vi "svx_Harmonic Generator.vi"(4 "noise amplitude":dbl=1.0 format="%.2f", 5 "# of harmonics":i32=5, 6 "sampling info":cluster{"Fs":dbl, "#s":dbl}={"Fs"=51200.0, "#s"=1024.0} {"#s" format="%.2p"; "Fs" format="%.2p"}, 7 "harmonics":T1(ring), 8 "error in (no error)":errorcluster, 9 "phase":dbl format="%.2f", 10 "Amplitude":dbl format="%.2f", 11 "fundamental":dbl format="%.2f") -> (0 "error out":errorcluster, 3 "Waveform":waveform(dbl))   [LabVIEW 2017]
uses:
  <vilib>/measure/maUtilsandCtls.llb/ma_Updatet0 DBL.vi
  <vilib>/measure/NI_MABase.lvlib
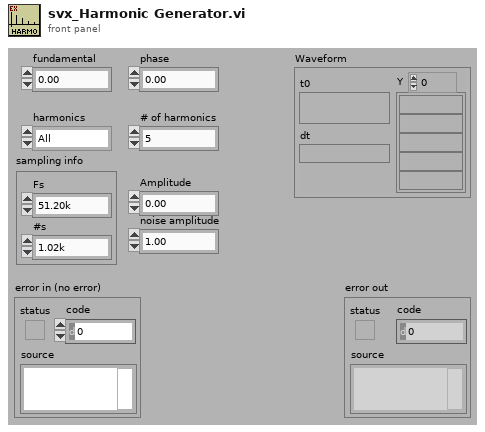
[diagram p1: front panel]
types:
  T1 = enum16{"All", "odd only", "even only", "Custom frequencies"}
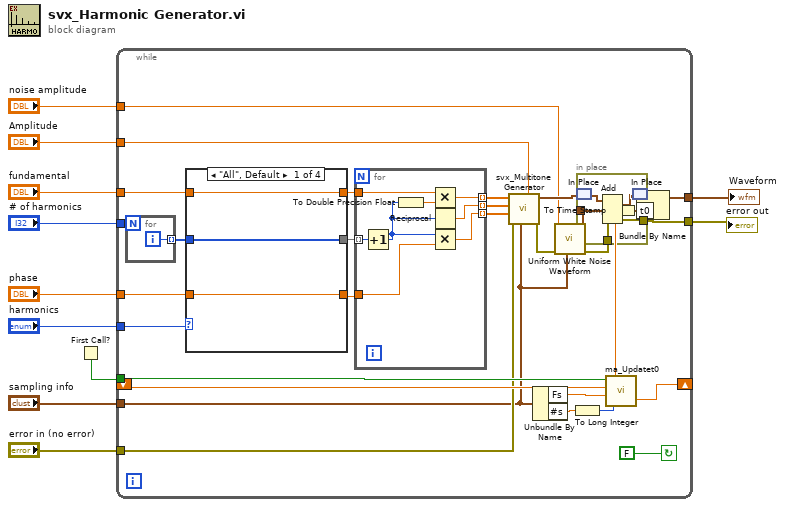
[diagram p0: block diagram]
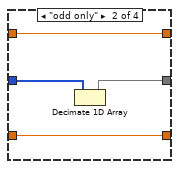
[diagram p2: hidden frame]
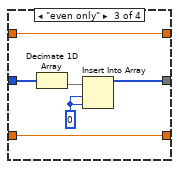
[diagram p3: hidden frame]
diagram:
  n1 = First Call?() -> (First Call?: T/F=w7:bool)
  n2 = while {
    tunnel: [w13] -> w1
    tunnel: "noise amplitude" -> [w14]
    tunnel: "error in (no error)" -> [w21]
    tunnel: "Amplitude" -> [w22]
    tunnel: w7 -> [w26]
    shift-left: _ -> [w28]
    shift-right: [w25] -> _
    tunnel: "phase" -> [w33]
    tunnel: [w27] -> w6
    tunnel: "fundamental" -> [w35]
    tunnel: "harmonics" -> [w40]
    tunnel: "# of harmonics" -> [w41]
    tunnel: "sampling info" -> [w15]
    stop <- FALSE continue-if-true
    n3 = for {
      N: w41 -> [_]
      tunnel: [w72] -> w38 mode=indexing
      i -> [w72]
    }
    n4 = case shown="\"All\", Default" w40 {
      tunnel: [w58 w62 w66 w71] -> w37
      tunnel: w38 -> [w58 w61 w65 w71]
      tunnel: w35 -> [w57 w60 w64 w70]
      tunnel: [w57 w60 w64 w70] -> w34
      tunnel: w33 -> [w56 w59 w63 w69]
      tunnel: [w56 w59 w63 w69] -> w32
      frame "All", Default {
      }
      frame "odd only" {
        n5 = Decimate 1D Array(w61) -> (w62:i32[])  [unwired: 1 out]
      }
      frame "even only" {
        w67 = 0 ("Index")
        n6 = Decimate 1D Array(w65) -> (w68:i32[])  [unwired: 1 out]
        n7 = Insert Into Array(array=w68, index=w67, new element=w67) -> (w66:i32[])
      }
      frame "Custom frequencies" {
        # "to be implemented"
      }
    }
    n8 = for {
      tunnel: w37 -> [w55] mode=indexing
      tunnel: w34 -> [w48]
      tunnel: [w54] -> w39 mode=indexing
      tunnel: w32 -> [w51]
      tunnel: [w50] -> w36 mode=indexing
      tunnel: [w53] -> w23 mode=indexing
      n9 = Increment(x=w55) -> (x+1=w52:i32)
      n10 = To Double Precision Float(number=w52) -> (double precision float=w49:dbl)
      n11 = Multiply(x=w48, y=w49) -> (x*y=w53:dbl)
      n12 = Reciprocal(x=w52) -> (1/x=w54:dbl)
      n13 = Multiply(x=w52, y=w51) -> (x*y=w50:dbl)
    }
    n14 = call <vilib>:"svx_Multitone Generator.vi"("amplitude"=w22, "sampling info"=w15, "error in (no error)"=w21, "tone phases"=w36, "tone amplitudes"=w39, "tone frequencies"=w23) -> ("error out"=w18:errorcluster, "signal out"=w20:waveform(dbl))  [unwired: 3 in, 1 out]
    n15 = Unbundle By Name(w15) -> ("Fs"=w31:dbl, "#s"=w30:dbl)
    n16 = call <vilib>:"Uniform White Noise Waveform.vi"("sampling info"=w15, "error in (no error)"=w18, "amplitude"=w14) -> ("error out"=w17:errorcluster, "signal out"=w16:waveform(dbl))  [unwired: 7 in]
    n17 = To Long Integer(number=w30) -> (32bit integer=w29:i32)
    n18 = in-place {
      in-place-border: w17 -> [w45]
      in-place-border: w16 -> [w44]
      in-place-border: [w43] -> w13
      n19 = in-place-match #1(w20) -> (w47:waveform(dbl))
      n20 = Add(1:w44, 2:w47, 4:w45) -> (0:w46:waveform(dbl), 3:w43:errorcluster)
      n21 = in-place-match #1(w46) -> (w19:waveform(dbl))
    }
    n22 = call-poly <vilib>:"ma_Updatet0.vi"("samples"=w29, "sampling rate (S/s)"=w31, "tf previous"=w28, "Reset Generation"=w26) -> ("tf new"=w25:dbl, "t0"=w24:dbl)
    n23 = To Time Stamp(1:w24) -> (0:w12:timestamp)
    n24 = Bundle By Name(cluster=w19, "t0"=w12) -> (w27:waveform(dbl))
  }
  "error out" <- w1
  "Waveform" <- w6
